vi "Static single axis example.vi"   [LabVIEW 2019]
uses:
  Axis Manager/Axis config.ctl
  Axis Manager/Axis enum.ctl
panel:
  # "Static single axis example\n\nOpen Block Diagram (ctrl-E)\nto see the code."
types:
  T1 = typedef "Axis config.ctl" = cluster{"Letter":string, "Stagetype":T2}
  T2 = typedef "Axis enum.ctl" = enum16{"XLA with 50 µm resolution", "XLA with 10 µm resolution", "XLA with 1250 nm resolution", "XLA with 312 nm resolution", "XLA with 78 nm resolution", "XLS with 1250 nm resolution", "XLS with 312 nm resolution", "XLS with 78nm resolution", "XLS with 5nm resolution", "XLS with 1 nm resolution", "XRT-A with 109 µrad resolution", "XRT-U-30 with 109 µrad resolution", "XRT-U-30 with 49 µrad resolution", "XRT-U-30 with 19 µrad resolution", "XRT-U-30 with 3 µrad resolution", "XRT-U-40 with 109 µrad resolution", "XRT-U 40 with 49 µrad resolution", "XRT-U-40 with 19 µrad resolution", "XRT-U-40 with 3 µrad resolution", "XRT-U-60 with 109 µrad resolution", "XRT-U-60 with 49 µrad resolution", "XRT-U-60 with 19 µrad resolution", "XRT-U-60 with 3 µrad resolution"}
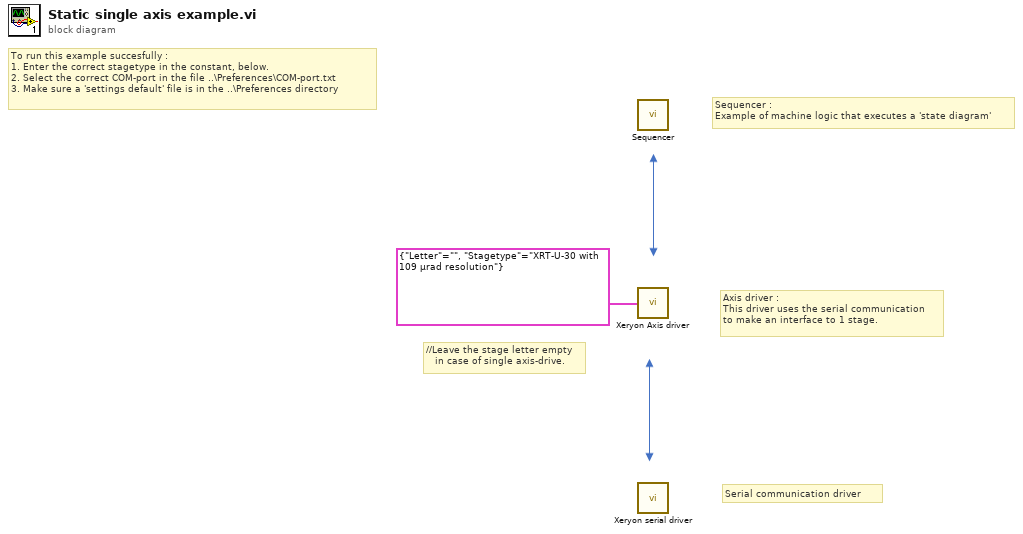
[diagram p0: block diagram]
diagram:
  # "To run this example succesfully :\n1. Enter the correct stagetype in the constant, below.\n2. Select the correct COM-port in the file ..\\Preferences\\COM-port.txt\n3. Make sure a 'settings default' file is in the ..\\Preferences directory"
  # "//Leave the stage letter empty\n   in case of single axis-drive."
  # "Sequencer :\nExample of machine logic that executes a 'state diagram'"
  # "Axis driver :\nThis driver uses the serial communication\nto make an interface to 1 stage."
  # "Serial communication driver"
  n1 = call "Sequencer.vi"() -> ()  [unwired: 12 in]
  n2 = call "Xeryon Axis driver.vi"("Config"=T1 {"Letter"="", "Stagetype"=enum."XRT-U-30 with 109 µrad resolution"}) -> ()  [unwired: 5 in]
  n3 = call "Xeryon serial driver.vi"() -> ()  [unwired: 6 in]
